vi "Fetch Waveforms.vi"(8 "error in":errorcluster, 11 "object in":refnum<class "Fetch Display CFG.lvclass">) -> (0 "error out":errorcluster, 2 "Last Waveforms":map{u8, waveform(dbl)}(c390), 3 "object out":refnum<class "Fetch Display CFG.lvclass">)   [LabVIEW 2023, in "RIGOL DS1054.lvlib" / "Fetch Display CFG.lvclass"]
uses:
  Fetch Display CFG.lvclass
  Scope VISA/Configuration/Scope VISA CFG.lvclass/Scope VISA CFG.ctl
  Configuration Base/Configuration Base.lvclass/Configuration Base.ctl
  8d36052f-398f-4416-96a9-5ca09e3acc97.vi
  ce682fe7-8147-45a0-826f-6225c648e612.vi
  02167e95-eb1b-459e-9628-7c497ad36d0b.vi
  <vilib>/JDP Science/JSONtext/Find Item.vi
  <vilib>/JDP Science/JSONtext/Next JSON Value.vi
  <vilib>/JDP Science/JSONtext/String Subset.vi
  <vilib>/JDP Science/JSONtext/Parsing/Advance past next JSON Value (inlined COPY).vi
  <vilib>/JDP Science/JSONtext/Parsing/Advance past whitespace.vi
  <vilib>/JDP Science/JSONtext/Parsing/Advance past String.vi
  <vilib>/JDP Science/JSONtext/Parsing/Advance past Number.vi
  <vilib>/JDP Science/JSONtext/Parsing/Advance past Line Ending.vi
  <vilib>/JDP Science/JSONtext/Parsing/Parse Full Path or Item Name.vi
  <vilib>/JDP Science/JSONtext/Parsing/Advance past Array.vi
  <vilib>/JDP Science/JSONtext/Parsing/Advance past Object.vi
  <vilib>/JDP Science/JSONtext/support/Error Cluster From Code.vi
  <vilib>/JDP Science/JSONtext/Offset/Find Item Locations by Path.vi
  <vilib>/JDP Science/JSONtext/JSON text to Variant.vi
  <vilib>/JDP Science/JSONtext/LVClass Serializer/JSONtext LVClass Serializer.lvclass
  Fetch Display CFG.lvclass/Fetch Display CFG.ctl
  Scope VISA/Configuration/Scope VISA CFG.lvclass
  Configuration Base/Configuration Base.lvclass
  RIGOL-DS1054Z-LabVIEW/RIGOL DS1054Z.lvlib
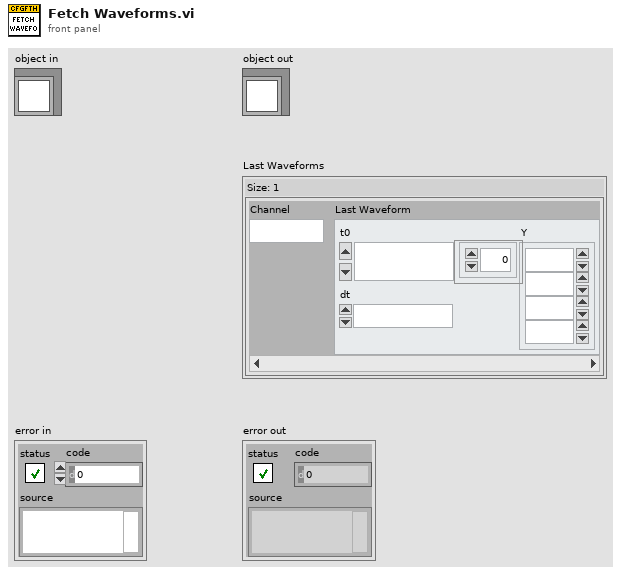
[diagram p1: front panel]
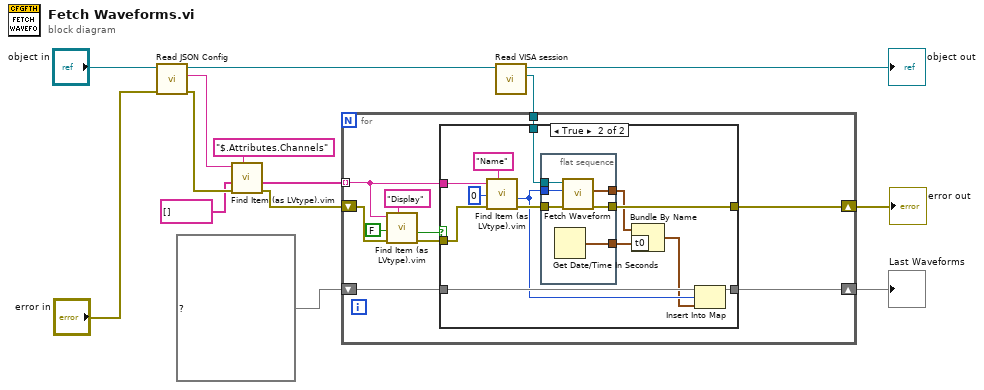
[diagram p0: block diagram]
diagram:
  n1 = call "Read JSON Config.vi"("error in (no error)"="error in", "object in"="object in") -> ("error out"=w12:errorcluster, "<JSON>Config"=w7:string, "object out"=w10:refnum<class "Fetch Display CFG.lvclass">)  [unwired: 7 in]
  n2 = call "Find Item (as LVtype).vim"("$Path or Item Name"="$.Attributes.Channels", "error in (no error)"=w12, "Data Type and Default Value"=string[] [], "JSON"=w7) -> ("error out"=w5:errorcluster, "Data"=w6:string[])  [unwired: 4 in, 2 out]
  n3 = call "Read VISA session.vi"("Scope VISA CFG in"=w10) -> ("VISA session"=w4:refnum<visa-resource-name>, "Scope VISA CFG out"=→"object out":refnum<class "Fetch Display CFG.lvclass">)  [unwired: 8 in, 1 out]
  n4 = for {
    tunnel: w6 -> [w19] mode=indexing
    tunnel: w4 -> [w18]
    shift-right: [w17] -> w1
    shift-left: w5 -> [w24]
    shift-right: [w15] -> w2
    shift-left: map{u8, waveform(dbl)} {} ("Last Waveforms") -> [w16]
    n5 = call "Find Item (as LVtype).vim"("$Path or Item Name"="Display", "error in (no error)"=w24, "Data Type and Default Value"=FALSE, "JSON"=w19) -> ("error out"=w21:errorcluster, "Data"=w20:bool)  [unwired: 4 in, 2 out]
    n6 = case shown="True" w20 {
      tunnel: w21 -> [w25 w38]
      tunnel: w19 -> [_ w39]
      tunnel: w18 -> [_ w35]
      tunnel: [w25 w33] -> w17
      tunnel: w16 -> [w26 w32]
      tunnel: [w26 w30] -> w15
      frame False {
      }
      frame True {
        n7 = call "Find Item (as LVtype).vim"("$Path or Item Name"="Name", "error in (no error)"=w38, "Data Type and Default Value"=u16 0, "JSON"=w39) -> ("error out"=w34:errorcluster, "Data"=w31:u16)  [unwired: 4 in, 2 out]
        n8 = flat-sequence {
          tunnel: w35 -> [w45]
          tunnel: w34 -> [w44]
          tunnel: [w43] -> w33
          tunnel: w31 -> [w40]
          tunnel: [w42] -> w29
          tunnel: [w41] -> w27
          frame #0 {
            n9 = Get Date/Time In Seconds() -> (seconds since 1Jan1904=w41:timestamp)
            n10 = call "Fetch Waveform.vi"("error in (no error)"=w44, "Channel (1: Channel 1)"=w40, "VISA resource name"=w45) -> ("error out"=w43:errorcluster, "Waveform Data"=w42:waveform(dbl))  [unwired: 6 in, 1 out]
          }
        }
        n11 = Bundle By Name(cluster=w29, "t0"=w27) -> (w28:waveform(dbl))
        n12 = Insert Into Map(map in=w32, key=w31, value=w28) -> (map out=w30:map{u8, waveform(dbl)})  [unwired: 2 out]
      }
    }
  }
  "error out" <- w1
  "Last Waveforms" <- w2
